vi "ReDraw ROI.vi"(6 "Mode (Redraw All)":enum16{"Redraw All", "Draw Last"}(ring), 8 "error in":errorcluster, 11 "XYZ Coordinates":T1[](array[typedef]) {"ROI group ID" format="%#_6f"; "Laser Power (%)" format="%#_6f"; "Zoom" format="%#_6f"; "Frame Size" format="%#_6f"; "Number of lines" format="%#_6f"; "Composite ID" format="%#_6f"; "Angle (deg)" format="%#_6f"; "ROI Time (ns)" format="%#_6f"; "ROI ID" format="%#_6f"; "Pixels in ROI" format="%#_6f"; "ROI index" format="%#_6f"; "Z stop" format="%#_6f"; "Y stop" format="%#_6f"; "X stop" format="%#_6f"; "Z start" format="%#_6f"; "X start" format="%#_6f"; "Y start" format="%#_6f"}) -> (0 "error out":errorcluster)   [LabVIEW 2013]
uses:
  Visualisation/Functional Imaging Viewer/Typedefs/ROI parameters data type.ctl
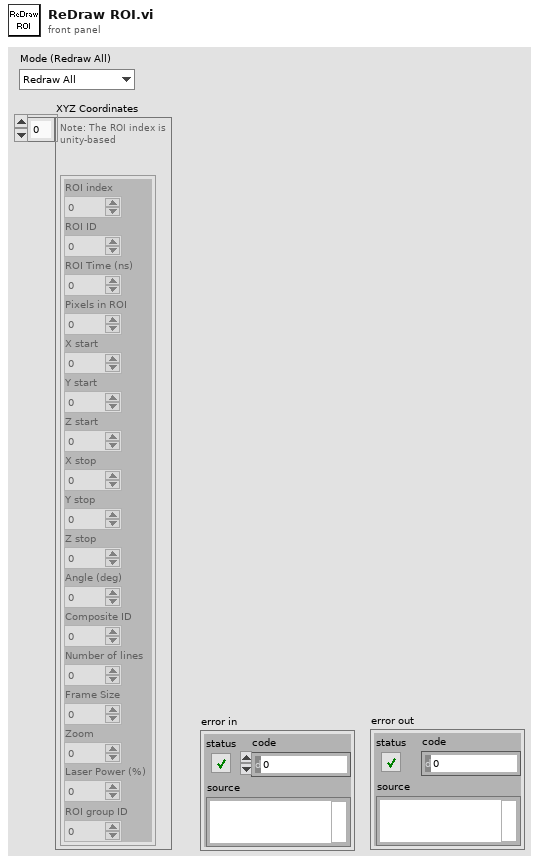
[diagram p1: front panel]
types:
  T1 = typedef "ROI parameters data type.ctl" = cluster{"ROI index":dbl, "ROI ID":dbl, "ROI Time (ns)":dbl, "Pixels in ROI":dbl, "X start":dbl, "Y start":dbl, "Z start":dbl, "X stop":dbl, "Y stop":dbl, "Z stop":dbl, "Angle (deg)":dbl, "Composite ID":dbl, "Number of lines":dbl, "Frame Size":dbl, "Zoom":dbl, "Laser Power (%)":dbl, "ROI group ID":dbl}
  T2 = typedef "IMAQ Image.ctl" = refnum<image>
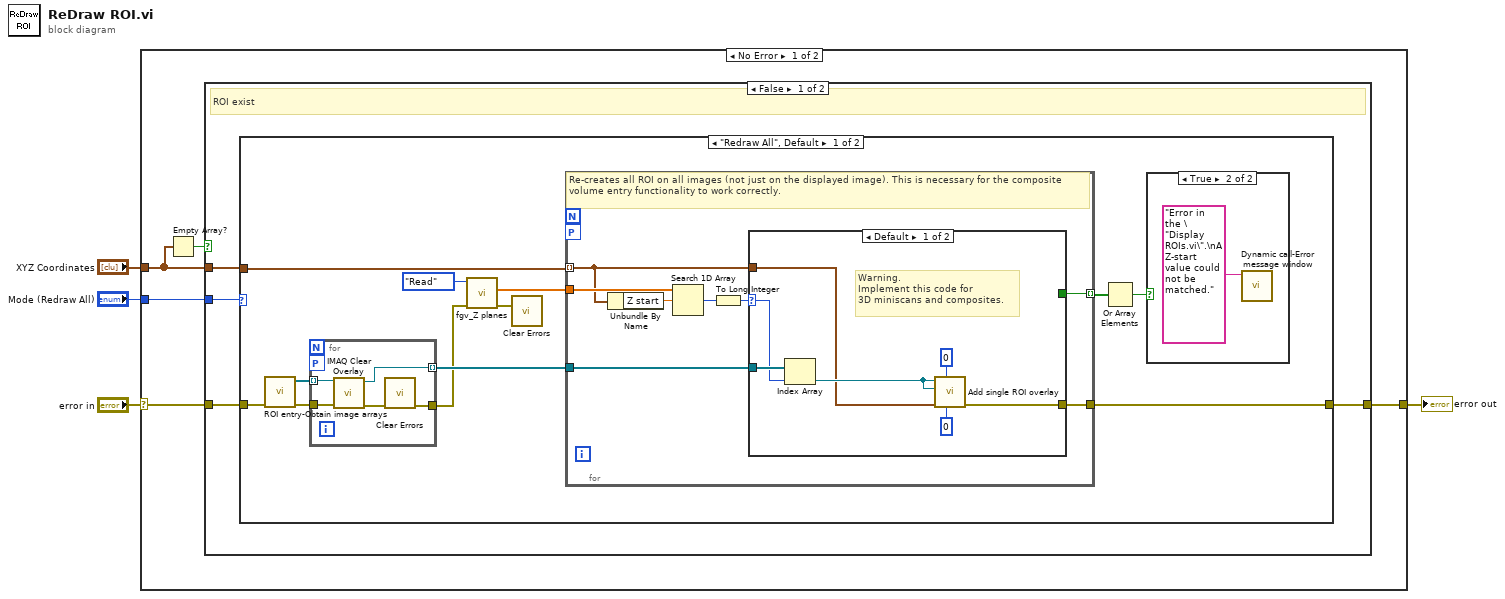
[diagram p0: block diagram]
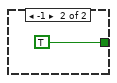
[diagram p3: hidden frame]
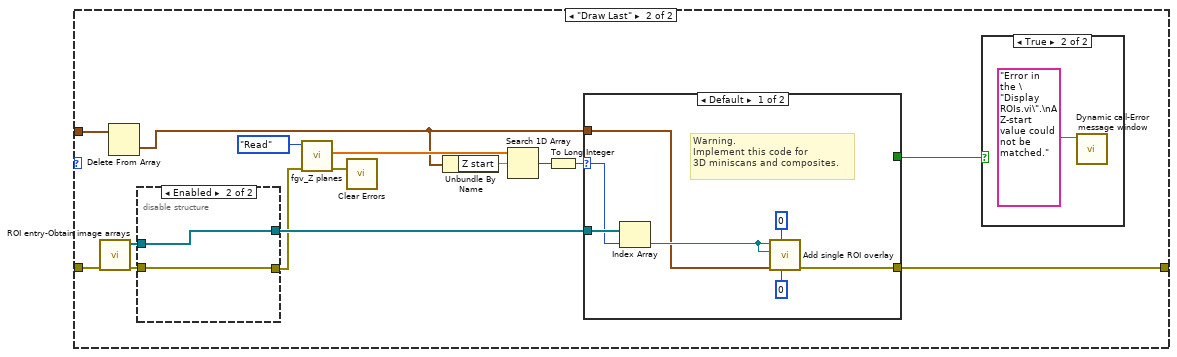
[diagram p4: hidden frame]
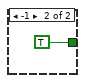
[diagram p5: hidden frame]
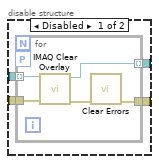
[diagram p6: hidden frame]
diagram:
  n1 = case shown="No Error" "error in" {
    selector: "error in" -> [w7 w84]
    tunnel: "XYZ Coordinates" -> [w9 _]
    tunnel: [w8 w84] -> w2
    tunnel: "Mode (Redraw All)" -> [w5 _]
    frame No Error {
      n2 = Empty Array?(array=w9) -> (empty?=w6:bool)
      n3 = case shown="False" w6 {
        tunnel: w9 -> [w13 _]
        tunnel: [w12 w83] -> w8
        tunnel: w7 -> [w11 w83]
        tunnel: w5 -> [w10 _]
        frame False {
          # "ROI exist"
          n4 = case shown="\"Redraw All\", Default" w10 {
            tunnel: w13 -> [w25 w53]
            tunnel: [w17 w57] -> w12
            tunnel: w11 -> [w14 w54]
            frame "Redraw All", Default {
              n5 = call "ROI entry-Obtain image arrays.vi"("error in (no error)"=w14) -> ("error IO"=w15:errorcluster, "RedImageArray"=w16:T2[])  [unwired: 9 in]
              n6 = for {
                tunnel: w16 -> [w31] mode=indexing
                tunnel: [w30] -> w24 mode=indexing
                workers-P: _ -> [_]
                tunnel: [w28] -> w19
                tunnel: w15 -> [w27]
                n7 = call "IMAQ Clear Overlay"("error in (no error)"=w27, "Image"=w31) -> ("error out"=w29:errorcluster, "Image Out"=w30:T2)  [unwired: 8 in]
                n8 = call <vilib>:"Clear Errors.vi"("error in (no error)"=w29) -> ("error out"=w28:errorcluster)  [unwired: 6 in]
              }
              n9 = call "fgv_Z planes.vi"("error in (no error)"=w19, "Function"=enum16{"Intialize", "Write", "Read", "Clear"}."Read") -> ("error out"=w18:errorcluster, "AOL Z Planes"=w22:dbl[])  [unwired: 7 in, 1 out]
              n10 = call <vilib>:"Clear Errors.vi"("error in (no error)"=w18) -> ()  [unwired: 6 in, 1 out]
              n11 = for {
                tunnel: w25 -> [w36] mode=indexing
                tunnel: w22 -> [w39]
                tunnel: w24 -> [w37]
                workers-P: _ -> [_]
                tunnel: [w33] -> w21 mode=indexing
                tunnel: [w32] -> w17
                # "Re-creates all ROI on all images (not just on the displayed image). This is necessary for the composite volume entry functionality to work correctly."
                n12 = Unbundle By Name(w36) -> ("Z start"=w38:dbl)
                n13 = Search 1D Array(1D array=w39, element=w38) -> (index of element=w35:i32)  [unwired: 1 in]
                n14 = To Long Integer(number=w35) -> (32bit integer=w34:i32)
                n15 = case shown="Default" w34 {
                  selector: w34 -> [w42 _]
                  tunnel: w37 -> [w46 _]
                  tunnel: w36 -> [w44 _]
                  tunnel: [_ TRUE] -> w33
                  tunnel: [w40 _] -> w32
                  frame Default {
                    # "Warning.\nImplement this code for\n3D miniscans and composites."
                    n16 = Index Array(array=w46, index=w42) -> (element=w45:T2)
                    n17 = call "Add single ROI overlay.vi"("Abs. index of selected Z-plane (unity-based)"=0, "Number of Z-planes"=0, "ROI Properties"=w44, "Image2"=w45, "Image1"=w45) -> ("Error out"=w40:errorcluster)  [unwired: 4 in, 2 out]
                  }
                  frame -1 {
                  }
                }
              }
              n18 = Or Array Elements(Boolean array=w21) -> (logical OR=w20:bool)
              n19 = case shown="True" w20 {
                frame False {
                }
                frame True {
                  n20 = call "Dynamic call-Error message window.vi"("Error Message"="Error in the \"Display ROIs.vi\".\nA Z-start value could not be matched.") -> ()  [unwired: 10 in, 1 out]
                }
              }
            }
            frame "Draw Last" {
              n21 = call "ROI entry-Obtain image arrays.vi"("error in (no error)"=w54) -> ("error IO"=w55:errorcluster, "RedImageArray"=w56:T2[])  [unwired: 9 in]
              n22 = Delete From Array(array=w53) -> (deleted portion=w52:T1)  [unwired: 2 in, 1 out]
              n23 = disable-structure shown="Enabled" {
                disable-tunnel: [w74 w81] -> w62
                disable-tunnel: [w73 w80] -> w59
                disable-tunnel: w56 -> [w72 w81]
                disable-tunnel: w55 -> [w71 w80]
                frame Disabled {
                  n24 = for {
                    tunnel: w72 -> [w79] mode=indexing
                    tunnel: [w78] -> w74 mode=indexing
                    workers-P: _ -> [_]
                    tunnel: [w76] -> w73
                    tunnel: w71 -> [w75]
                    n25 = call "IMAQ Clear Overlay"("error in (no error)"=w75, "Image"=w79) -> ("error out"=w77:errorcluster, "Image Out"=w78:T2)  [unwired: 8 in]
                    n26 = call <vilib>:"Clear Errors.vi"("error in (no error)"=w77) -> ("error out"=w76:errorcluster)  [unwired: 6 in]
                  }
                }
                frame Enabled {
                }
              }
              n27 = call "fgv_Z planes.vi"("error in (no error)"=w59, "Function"=enum16{"Intialize", "Write", "Read", "Clear"}."Read") -> ("error out"=w58:errorcluster, "AOL Z Planes"=w60:dbl[])  [unwired: 7 in, 1 out]
              n28 = call <vilib>:"Clear Errors.vi"("error in (no error)"=w58) -> ()  [unwired: 6 in, 1 out]
              n29 = Unbundle By Name(w52) -> ("Z start"=w51:dbl)
              n30 = Search 1D Array(1D array=w60, element=w51) -> (index of element=w50:i32)  [unwired: 1 in]
              n31 = To Long Integer(number=w50) -> (32bit integer=w49:i32)
              n32 = case shown="Default" w49 {
                selector: w49 -> [w65 _]
                tunnel: w62 -> [w69 _]
                tunnel: w52 -> [w67 _]
                tunnel: [_ TRUE] -> w48
                tunnel: [w63 _] -> w57
                frame Default {
                  # "Warning.\nImplement this code for\n3D miniscans and composites."
                  n33 = Index Array(array=w69, index=w65) -> (element=w68:T2)
                  n34 = call "Add single ROI overlay.vi"("Abs. index of selected Z-plane (unity-based)"=0, "Number of Z-planes"=0, "ROI Properties"=w67, "Image2"=w68, "Image1"=w68) -> ("Error out"=w63:errorcluster)  [unwired: 4 in, 2 out]
                }
                frame -1 {
                }
              }
              n35 = case shown="True" w48 {
                frame False {
                }
                frame True {
                  n36 = call "Dynamic call-Error message window.vi"("Error Message"="Error in the \"Display ROIs.vi\".\nA Z-start value could not be matched.") -> ()  [unwired: 10 in, 1 out]
                }
              }
            }
          }
        }
        frame True {
          # "ROI array is empty"
        }
      }
    }
    frame Error {
    }
  }
  "error out" <- w2
